vi "Format Integer Tables.vi"(0 "Header":string[](array[string]), 5 "Data Table":dbl[][](array[numeric])) -> (4 "spreadsheet string":string)   [LabVIEW 2010]
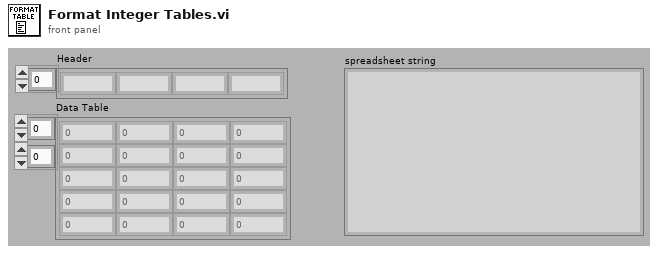
[diagram p1: front panel]
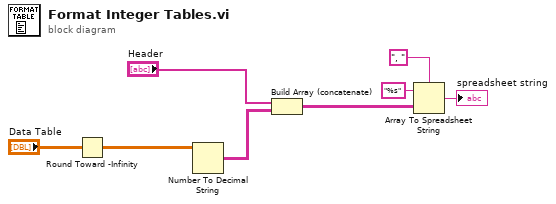
[diagram p0: block diagram]
diagram:
  n1 = Round Toward -Infinity(1:"Data Table") -> (0:w1:dbl[][])
  n2 = Number To Decimal String(number=w1) -> (decimal integer string=w7:string[][])  [unwired: 1 in]
  n3 = Build Array (concatenate)("Header", w7) -> (w6:string[][])
  n4 = Array To Spreadsheet String(delimiter (Tab)=", ", array=w6, 3:"%s" ("format string")) -> (spreadsheet string=→"spreadsheet string":string)
